vi "GeneralHandler.vi"(5 "[user-defined descriptions]":string[](array[string]), 7 "[user-defined codes]":i32[](array[numeric]), 8 "error in (no error)":errorcluster) -> (0 "Severity":string, 1 "Stop":bool, 2 "Abort":bool, 3 "Continue":bool)   [LabVIEW 2014, in "NISTErrorLib.lvlib"]
uses:
  NISTErrorLib.lvlib
  eDialogType.ctl
  <vilib>/Utility/error.llb/whitespace.ctl
panel:
  in  "String to Format (not a refnum)":refnum<vi>
  # "The General handler currently looks for the following severities:\n\n     Fatal  \n     Critical\n     Abort (when a process or state machine needs to stop but the application can continue.\n     Warning\n     Inform\n     Log (no dialog will be launched)"
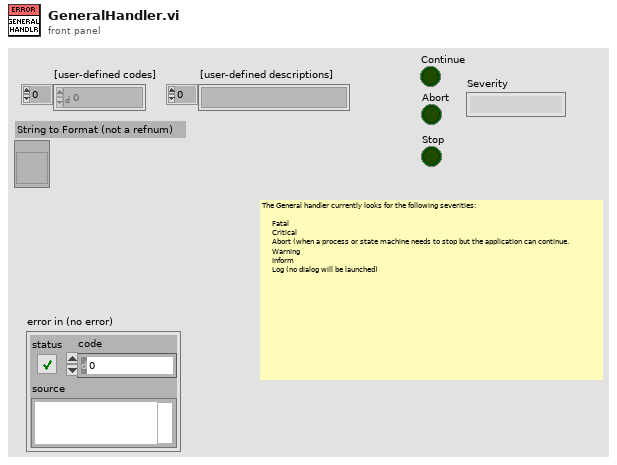
[diagram p1: front panel]
types:
  T1 = enum16{"no dialog", "Continue", "Continue Stop", "Abort Continue Stop", "Stop"}
  T2 = typedef "NISTErrorLib.lvlib/eDialogType.ctl" = enum16{"no dialog", "Continue", "Continue Stop", "Abort Continue Stop", "Stop"}
  T3 = typedef "TagReturnType.ctl" = enum16{"No Tag", "<err>", "<append>"}
  T4 = typedef "whitespace.ctl" = u16
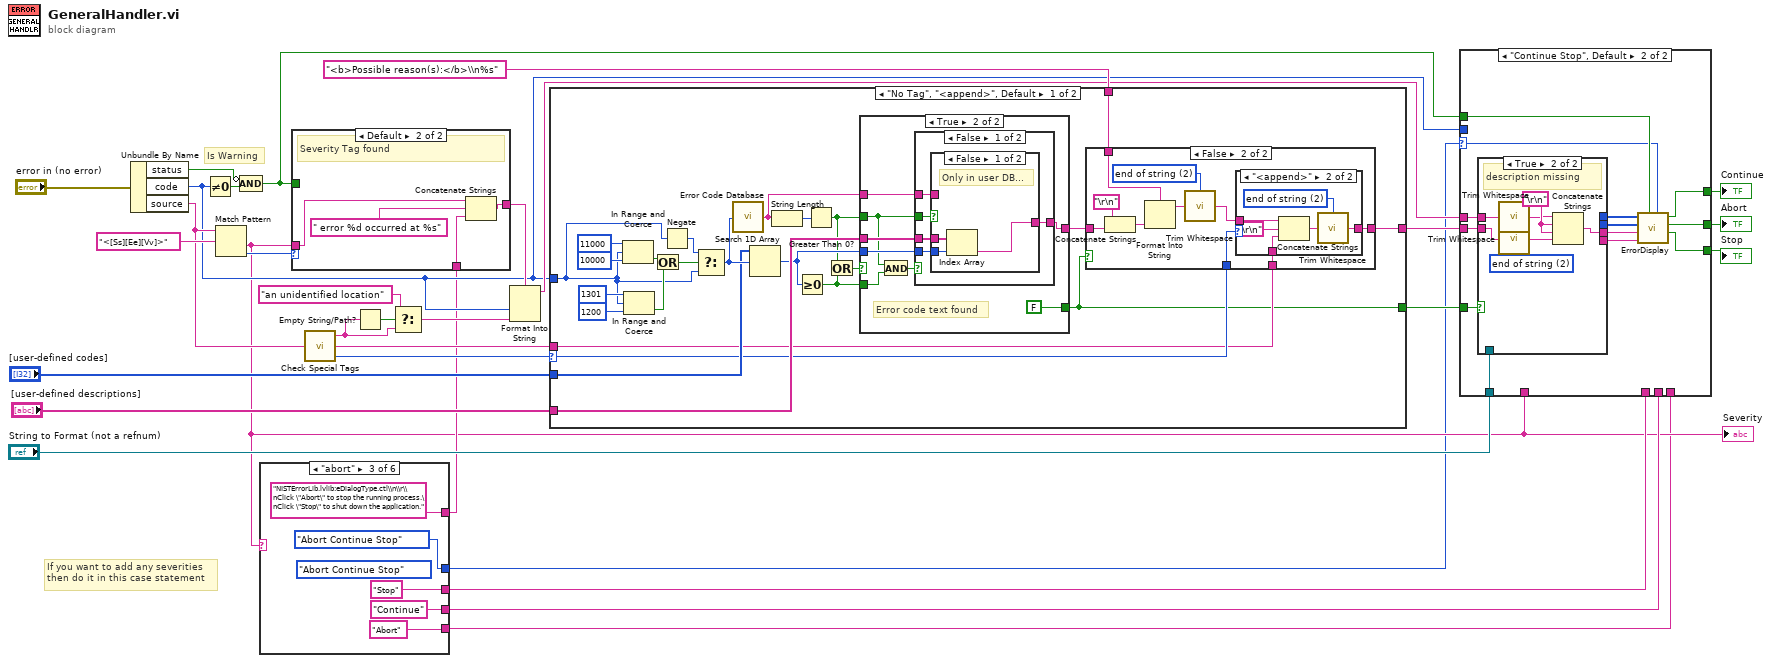
[diagram p0: block diagram]
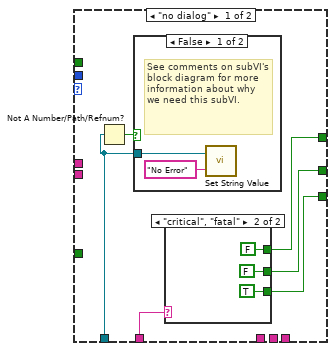
[diagram p2: hidden frame]
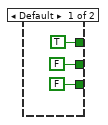
[diagram p3: hidden frame]
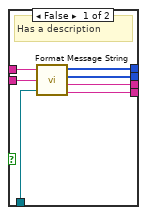
[diagram p5: hidden frame]
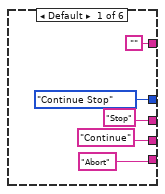
[diagram p6: hidden frame]
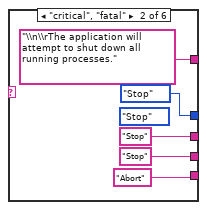
[diagram p7: hidden frame]
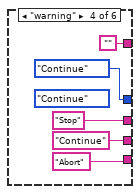
[diagram p8: hidden frame]
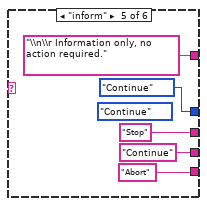
[diagram p9: hidden frame]
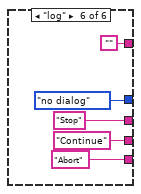
[diagram p10: hidden frame]
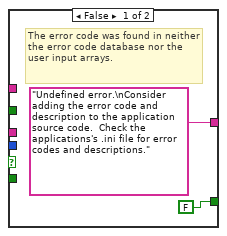
[diagram p13: hidden frame]
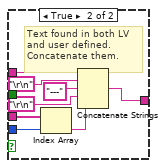
[diagram p15: hidden frame]
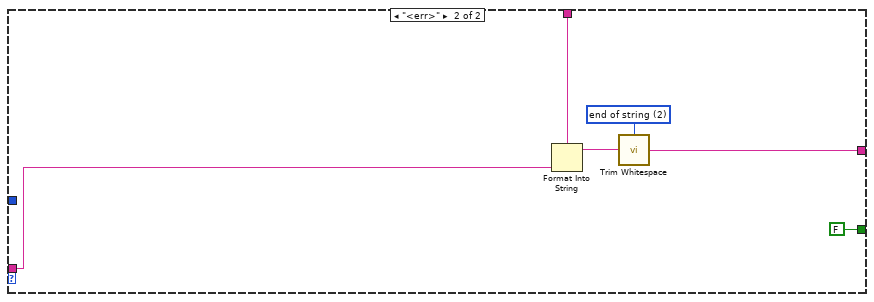
[diagram p16: hidden frame]
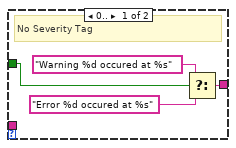
[diagram p17: hidden frame]
diagram:
  # "If you want to add any severities\nthen do it in this case statement"
  # "Is Warning"
  n1 = Unbundle By Name("error in (no error)") -> ("status"=w29:bool, "code"=w11:i32, "source"=w26:string)
  n2 = Not Equal To 0?(x=w11) -> (x != 0?=w30:bool)
  n3 = Match Pattern(string=w26, regular expression="<[Ss][Ee][Vv]>") -> (after substring=w5:string, offset past match=w27:i32)  [unwired: 1 in, 2 out]
  "Severity" <- w5
  n4 = Compound Arithmetic op=AND(invert w29, w30) -> (w12:bool)
  n5 = case shown="\"abort\"" w5 {
    tunnel: ["Stop" "Stop" "Stop" "Stop" "Stop" "Stop"] -> w10
    tunnel: ["Continue" "Stop" "Continue" "Continue" "Continue" "Continue"] -> w9
    tunnel: ["" "\\n\\rThe application will attempt to shut down all running processes." "NISTErrorLib.lvlib:eDialogType.ctl\\n\\r\\nClick \"Abort\" to stop the running process.\nClick \"Stop\" to shut down the application." "" "\\n\\r Information only, no action required." ""] -> w7
    tunnel: ["Abort" "Abort" "Abort" "Abort" "Abort" "Abort"] -> w4
    tunnel: [T1."Continue Stop" ("eDialogType") eDialogType."Stop" ("eDialogType") eDialogType."Abort Continue Stop" ("eDialogType") eDialogType."Continue" ("eDialogType") eDialogType."Continue" ("eDialogType") eDialogType."no dialog" ("eDialogType")] -> w3
    frame Default {
    }
    frame "critical", "fatal" {
      (unwired) T1."Stop" ("eDialogType")
    }
    frame "abort" {
      (unwired) T1."Abort Continue Stop" ("eDialogType")
    }
    frame "warning" {
      (unwired) T1."Continue" ("eDialogType")
    }
    frame "inform" {
      (unwired) T1."Continue" ("eDialogType")
    }
    frame "log" {
    }
  }
  n6 = case shown="Default" w27 {
    tunnel: w12 -> [w63 _]
    tunnel: [w62 w67] -> w22
    tunnel: w5 -> [_ w69]
    tunnel: w7 -> [_ w66]
    frame 0.. {
      # "No Severity Tag"
      n7 = Select(t="Warning %d occured at %s", s=w63, f="Error %d occured at %s") -> (s? t:f=w62:string)
    }
    frame Default {
      # "Severity Tag found"
      n8 = Concatenate Strings(w69, " error %d occurred at %s" ("string"), w66) -> (w67:string)
    }
  }
  n9 = call <vilib>:"Check Special Tags.vi"("source"=w26) -> ("Before Tag (source)"=w23:string, "After Tag (special data)"=w20:string, "Tag Found?"=w8:T3)
  n10 = Empty String/Path?(string/path=w23) -> (empty?=w25:bool)
  n11 = Select(t="an unidentified location", s=w25, f=w23) -> (s? t:f=w21:string)
  n12 = Format Into String(format string=w22, w11, w21) -> (resulting string=w14:string)  [unwired: 2 in, 1 out]
  n13 = case shown="\"No Tag\", \"<append>\", Default" w8 {
    selector: w8 -> [w73 _]
    tunnel: w20 -> [w72 w143]
    tunnel: "<b>Possible reason(s):</b>\\n%s" -> [w74 w144]
    tunnel: [w71 w140] -> w15
    tunnel: w11 -> [w76 _]
    tunnel: "[user-defined codes]" -> [w82 _]
    tunnel: "[user-defined descriptions]" -> [w81 _]
    tunnel: [w70 FALSE] -> w16
    frame "No Tag", "<append>", Default {
      n14 = In Range and Coerce(upper limit=11000, x=w76, lower limit=10000) -> (In Range?=w91:bool)  [unwired: 1 out]
      n15 = In Range and Coerce(upper limit=1301, x=w76, lower limit=1200) -> (In Range?=w90:bool)  [unwired: 1 out]
      n16 = Or(x=w91, y=w90) -> (x .or. y?=w92:bool)
      n17 = Negate(x=w76) -> (-x=w86:i32)
      n18 = Select(t=w86, s=w92, f=w76) -> (s? t:f=w83:i32)
      n19 = call <vilib>:"Error Code Database.vi"("Error Code"=w83) -> ("Error Text"=w84:string)
      n20 = Search 1D Array(1D array=w82, element=w83) -> (index of element=w80:i32)  [unwired: 1 in]
      n21 = String Length(string=w84) -> (length=w85:i32)
      n22 = Greater Or Equal To 0?(x=w80) -> (x >= 0?=w78:bool)
      n23 = Greater Than 0?(x=w85) -> (x > 0?=w77:bool)
      n24 = Or(x=w77, y=w78) -> (x .or. y?=w79:bool)
      n25 = case shown="True" w79 {
        tunnel: w80 -> [_ w117]
        tunnel: ["Undefined error.\nConsider adding the error code and description to the application source code.  Check the applications's .ini file for error codes and descriptions." w115] -> w75
        tunnel: [FALSE FALSE] -> w70
        tunnel: w77 -> [_ w114]
        tunnel: w78 -> [_ w119]
        tunnel: w81 -> [_ w118]
        tunnel: w84 -> [_ w116]
        frame False {
          # "The error code was found in neither the error code database nor the user input arrays."
        }
        frame True {
          # "Error code text found"
          n26 = And(x=w114, y=w119) -> (x .and. y?=w120:bool)
          n27 = case shown="False" w120 {
            tunnel: w118 -> [w123 w138]
            tunnel: w117 -> [w122 w137]
            tunnel: w116 -> [w124 w131]
            tunnel: [w125 w135] -> w115
            tunnel: w114 -> [w126 _]
            frame False {
              n28 = case shown="False" w126 {
                tunnel: [w127 w130] -> w125
                tunnel: w124 -> [_ w130]
                tunnel: w123 -> [w129 _]
                tunnel: w122 -> [w128 _]
                frame False {
                  # "Only in user DB..."
                  n29 = Index Array(array=w129, index=w128) -> (element=w127:string)
                }
                frame True {
                  # "Only in LV DB..."
                }
              }
            }
            frame True {
              # "Text found in both LV\nand user defined. \nConcatenate them."
              n30 = Index Array(array=w138, index=w137) -> (element=w136:string)
              n31 = Concatenate Strings(w131, "\r\n" ("End of Line Constant"), "---" ("string"), "\r\n" ("End of Line Constant"), w136) -> (w135:string)
            }
          }
        }
      }
      n32 = case shown="False" w70 {
        tunnel: w74 -> [_ w104]
        tunnel: [w94 w96] -> w71
        tunnel: w75 -> [w94 w101]
        tunnel: w73 -> [_ w98]
        tunnel: w72 -> [_ w97]
        frame True {
          # "no explanation given for error."
        }
        frame False {
          w95 = T4 2 items=["both", "start of string", "end of string"] ("location (both)")
          n33 = Concatenate Strings("\r\n" ("End of Line Constant"), w101) -> (w102:string)
          n34 = Format Into String(format string=w104, w102) -> (resulting string=w103:string)  [unwired: 2 in, 1 out]
          n35 = call <vilib>:"Trim Whitespace.vi"("string"=w103, "location (both)"=w95) -> ("trimmed string"=w99:string)
          n36 = case shown="\"<append>\"" w98 {
            tunnel: w99 -> [w105 w110]
            tunnel: [w105 w107] -> w96
            tunnel: w97 -> [_ w109]
            frame "No Tag", Default {
            }
            frame "<append>" {
              w106 = T4 2 items=["both", "start of string", "end of string"] ("location (both)")
              n37 = Concatenate Strings(w110, "\r\n" ("End of Line Constant"), w109) -> (w108:string)
              n38 = call <vilib>:"Trim Whitespace.vi"("string"=w108, "location (both)"=w106) -> ("trimmed string"=w107:string)
            }
          }
        }
      }
    }
    frame "<err>" {
      w142 = T4 2 items=["both", "start of string", "end of string"] ("location (both)")
      n39 = Format Into String(format string=w144, w143) -> (resulting string=w141:string)  [unwired: 2 in, 1 out]
      n40 = call <vilib>:"Trim Whitespace.vi"("string"=w141, "location (both)"=w142) -> ("trimmed string"=w140:string)
    }
  }
  n41 = case shown="\"Continue Stop\", Default" w3 {
    selector: w3 -> [_ w159]
    tunnel: w16 -> [_ w171]
    tunnel: w15 -> [_ w170]
    tunnel: w14 -> [_ w169]
    tunnel: "String to Format (not a refnum)" -> [w149 w168]
    tunnel: w12 -> [_ w163]
    tunnel: w11 -> [_ _]
    tunnel: w10 -> [_ _]
    tunnel: w9 -> [_ _]
    tunnel: [w145 w162] -> w6
    tunnel: w5 -> [w148 _]
    tunnel: w4 -> [_ _]
    tunnel: [w146 w161] -> w2
    tunnel: [w147 w160] -> w1
    frame "no dialog" {
      n42 = Not A Number/Path/Refnum?(number/path/refnum=w149) -> (NaN/Path/Refnum?=w150:bool)
      n43 = case shown="False" w150 {
        tunnel: w149 -> [w158 _]
        frame False {
          # "See comments on subVI's block diagram for more information about why we need this subVI."
          n44 = call <vilib>:"Set String Value.vi"("No Error"="No Error", "String to Format (not a refnum)"=w158) -> ()
        }
        frame True {
        }
      }
      n45 = case shown="\"critical\", \"fatal\"" w148 {
        tunnel: [FALSE TRUE] -> w147
        tunnel: [TRUE FALSE] -> w146
        tunnel: [FALSE FALSE] -> w145
        frame Default {
        }
        frame "critical", "fatal" {
        }
      }
    }
    frame "Continue Stop", Default {
      n46 = case shown="True" w171 {
        tunnel: w170 -> [w178 w184]
        tunnel: w169 -> [w177 w185]
        tunnel: w168 -> [w176 _]
        tunnel: [w175 _] -> w164
        tunnel: [w174 _] -> w165
        tunnel: [w173 w179] -> w166
        tunnel: [w172 _] -> w167
        frame False {
          # "Has a description"
          n47 = call <vilib>:"Format Message String.vi"("Source"=w177, "Details"=w178, "String to Format (not a refnum)"=w176) -> ("Bold Start"=w175:i32[], "Bold Length"=w174:i32[], "Source Out"=w173:string, "Details Out"=w172:string)  [unwired: 1 in, 1 out]
        }
        frame True {
          w182 = "\r\n" ("End of Line Constant")
          w183 = T4 2 items=["both", "start of string", "end of string"] ("location (both)")
          # "description missing"
          n48 = call <vilib>:"Trim Whitespace.vi"("string"=w185, "location (both)"=w183) -> ("trimmed string"=w181:string)
          n49 = call <vilib>:"Trim Whitespace.vi"("string"=w184, "location (both)"=w183) -> ("trimmed string"=w180:string)
          n50 = Concatenate Strings(w181, w182, w182, w180) -> (w179:string)
        }
      }
      n51 = call "ErrorDisplay.vi"("eDialogType"=w159, "Warning (f)"=w163, "Details"=w167, "Source"=w166, "Length"=w165, "Start"=w164) -> ("bStop"=w160:bool, "bAbort"=w162:bool, "bContinue"=w161:bool)  [unwired: 3 in]
    }
  }
  "Abort" <- w6
  "Continue" <- w2
  "Stop" <- w1
